vi "Acoustic Weighting.vi"(0 "Spectrum":dbl[](array[numeric]), 2 "dF (Hz)":dbl=1.0, 3 "F0 (Hz)":dbl, 5 "Spectrum Mag Type":T1, 7 "Acoustic Weighting":T2) -> (14 "Weighted Spectrum":dbl[](array[numeric]))   [LabVIEW 2022 SP3, in "GSwFormDSP.lvclass"]
uses:
  GSwFormDSP.lvclass
  functions/Acoustic Weighting.ctl
  functions/Spectrum Mag Type.ctl
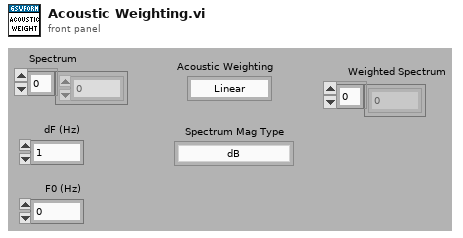
[diagram p1: front panel]
types:
  T1 = typedef "GSwFormDSP.lvclass/Spectrum Mag Type.ctl" = enum16{"dB", "EU", "EU²"}
  T2 = typedef "GSwFormDSP.lvclass/Acoustic Weighting.ctl" = enum16{"Linear", "A-weighting"}
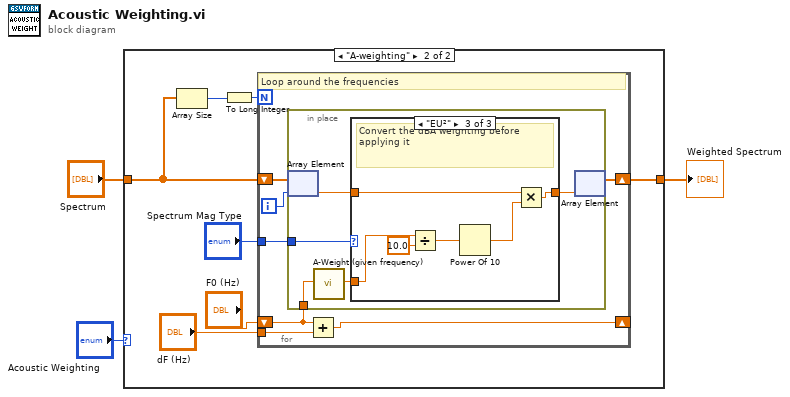
[diagram p0: block diagram]
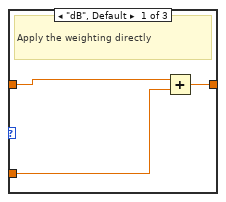
[diagram p3: hidden frame]
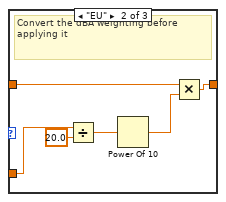
[diagram p4: hidden frame]
diagram:
  n1 = case shown="\"A-weighting\"" "Acoustic Weighting" {
    tunnel: [w4 w8] -> w3
    tunnel: "Spectrum" -> [w4 w7]
    frame "Linear", Default {
    }
    frame "A-weighting" {
      n2 = Array Size(array=w7) -> (size(s)=w6:i32)
      n3 = To Long Integer(number=w6) -> (32bit integer=w11:i32)
      n4 = for {
        N: w11 -> [_]
        shift-right: [w17] -> _
        shift-left: "F0 (Hz)" -> [w14]
        tunnel: "dF (Hz)" -> [w18]
        shift-right: [w13] -> w8
        shift-left: w7 -> [w16]
        tunnel: "Spectrum Mag Type" -> [w12]
        i -> [w15]
        # "Loop around the frequencies"
        n5 = in-place {
          in-place-border: w14 -> [w22]
          in-place-border: w12 -> [w19]
          n6 = in-place-array #1(w16, w15) -> (w23:dbl)
          n7 = call "A-Weight (given frequency).vi"("Frequency (Hz)"=w22) -> ("A-Weight (dB)"=w21:dbl)  [unwired: 18 in]
          n8 = case shown="\"EU²\"" w19 {
            tunnel: w23 -> [w26 w28 w34]
            tunnel: w21 -> [w25 w30 w36]
            tunnel: [w24 w29 w35] -> w20
            frame "dB", Default {
              # "Apply the weighting directly"
              n9 = Add(x=w26, y=w25) -> (x+y=w24:dbl)
            }
            frame "EU" {
              # "Convert the dBA weighting before  applying it"
              n10 = Divide(x=w30, y=20.0) -> (x/y=w31:dbl)
              n11 = Power Of 10(x=w31) -> (10^x=w27:dbl)
              n12 = Multiply(x=w28, y=w27) -> (x*y=w29:dbl)
            }
            frame "EU²" {
              # "Convert the dBA weighting before  applying it"
              n13 = Divide(x=w36, y=10.0) -> (x/y=w37:dbl)
              n14 = Power Of 10(x=w37) -> (10^x=w33:dbl)
              n15 = Multiply(x=w34, y=w33) -> (x*y=w35:dbl)
            }
          }
          n16 = in-place-array #1(w20) -> (w13:dbl[])  [unwired: 1 out]
        }
        n17 = Add(x=w14, y=w18) -> (x+y=w17:dbl)
      }
    }
  }
  "Weighted Spectrum" <- w3
